vi "sendMessage.vi"(8 "error in (no error)":errorcluster, 10 "String":string, 11 "TCPClient in":refnum<class "TCPClient.lvclass">) -> (0 "error out":errorcluster, 3 "TCPClient out":refnum<class "TCPClient.lvclass">)   [LabVIEW 2016, in "TCPClient.lvclass"]
uses:
  TCPClient.lvclass
  TCPSettings/TCPSettings.lvclass
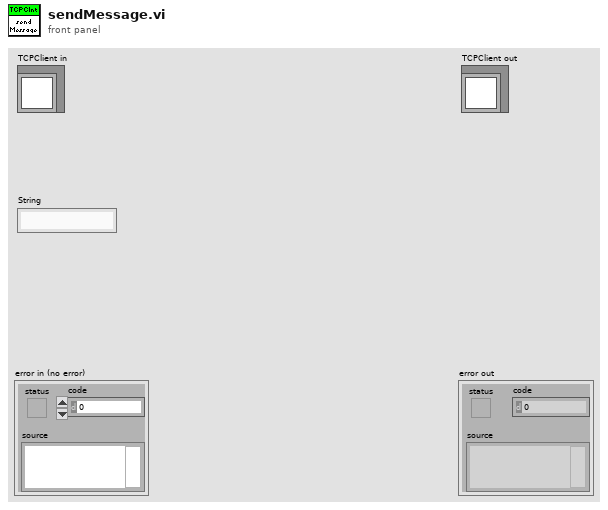
[diagram p1: front panel]
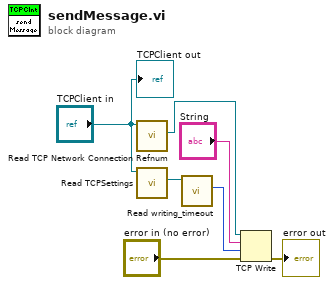
[diagram p0: block diagram]
diagram:
  n1 = call-dynamic "Read TCP Network Connection Refnum.vi"("TCPCommunicator in"="TCPClient in") -> ("TCP Network Connection Refnum"=w6:refnum<k5>)  [unwired: 8 in, 2 out]
  n2 = call-dynamic "Read TCPSettings.vi"("TCPCommunicator in"="TCPClient in") -> ("TCPSettings.lvclass"=w5:refnum<class "TCPSettings.lvclass">)  [unwired: 8 in, 2 out]
  n3 = call-dynamic "Read writing_timeout.vi"("TCPSettings in"=w5) -> ("writing_timeout"=w7:i32)  [unwired: 8 in, 2 out]
  n4 = TCP Write(connection ID=w6, data in="String", error in (no error)="error in (no error)", 9:w7) -> (error out=→"error out":errorcluster)  [unwired: 2 out]
  "TCPClient out" <- "TCPClient in"
